vi "Send View Front Panel.vi"(8 "error in (no error)":errorcluster, 10 "SubPnl Refnum":refnum<vi>, 11 "Message Enqueuer":refnum<class "Message Enqueuer.lvclass">) -> (0 "error out":errorcluster, 3 "Message Enqueuer out":refnum<class "Message Enqueuer.lvclass">)   [LabVIEW 2013, in "PluginInterface.lvlib" / "View Front Panel Msg.lvclass"]
uses:
  View Front Panel Msg.lvclass
  Actor Framework/Actor Framework.lvlibp/Message Enqueuer/Message Enqueuer.lvclass
  Actor Framework/Actor Framework.lvlibp/Message Enqueuer/Message Priority.ctl
  View Front Panel Msg.lvclass/View Front Panel Msg.ctl
panel:
  in  "Message Priority (Normal)":T1=enum."Normal"
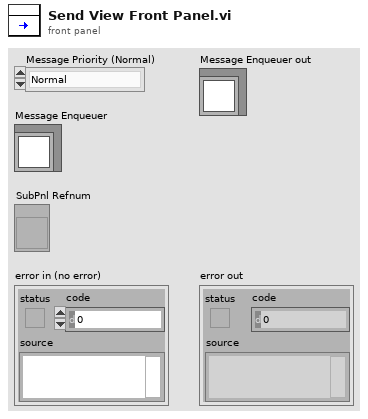
[diagram p1: front panel]
types:
  T1 = typedef "Actor Framework.lvlibp/Message Enqueuer.lvclass/Message Priority.ctl" = enum16{"Low", "Normal", "High"}
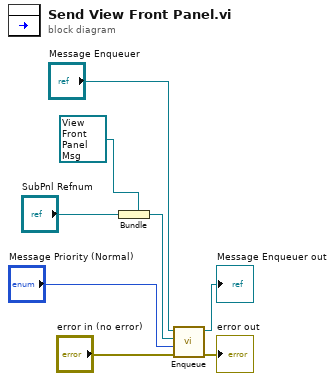
[diagram p0: block diagram]
diagram:
  n1 = Bundle(cluster=refnum<class "View Front Panel Msg.lvclass"> refnum ("PluginInterface.lvlib:View Front Panel Msg.lvclass"), "SubPnl Refnum") -> (w6:refnum<class "View Front Panel Msg.lvclass">)
  n2 = call "Enqueue.vi"("error in (no error)"="error in (no error)", "Message Priority (Normal)"="Message Priority (Normal)", "Message"=w6, "Message Enqueuer in"="Message Enqueuer") -> ("error out"=→"error out":errorcluster, "Message Enqueuer out"=→"Message Enqueuer out":refnum<class "Message Enqueuer.lvclass">)  [unwired: 6 in]
